vi "LSMcontroller_v65_updatedsealtest.vi"() -> ()   [LabVIEW 2015] (continued)
                                n2574 = call "tempconfigAO_seal.vi"("command"="get") -> ("Temp Config out"=w5707:T25)  [unwired: 1 in]
                                n2575 = Bundle By Name(cluster=w5707, "AO"=w5706, "E_AO"=w5705) -> (w5704:T25)
                                n2576 = call "tempconfigAO_seal.vi"("Temp Config in"=w5704, "command"="set") -> ()  [unwired: 1 out]
                                }
                                frame #1 {
                                n2577 = call "tempconfigAI_seal.vi"("command"="get") -> ("Temp Config out"=w5719:T26)  [unwired: 1 in]
                                n2578 = Unbundle By Name(w5719) -> ("AI"=w5724:refnum<k21>, "E_AI"=w5725:errorcluster)
                                n2579 = call <vilib>:"DAQmx Start Task.vi"("task/channels in"=w5724, "error in"=w5725) -> ("task out"=w5726:refnum<k21>, "error out"=w5727:errorcluster)  [unwired: 12 in]
                                n2580 = call "tempconfigAI_seal.vi"("command"="get") -> ("Temp Config out"=w5721:T26)  [unwired: 1 in]
                                n2581 = Bundle By Name(cluster=w5721, "AI"=w5726, "E_AI"=w5727) -> (w5723:T26)
                                n2582 = call "tempconfigAI_seal.vi"("Temp Config in"=w5723, "command"="set") -> ()  [unwired: 1 out]
                                }
                              }
                            }
                          }
                          n2583 = case shown="True" w5703 {
                            frame False {
                            }
                            frame True {
                              n2584 = local write "set as Rp?"(FALSE ("set as Rp?")) -> ()
                            }
                          }
                        }
                      }
                      n2585 = local read "sealtest"() -> (w5590:bool)
                      n2586 = Not(x=w5590) -> (.not. x?=w5589:bool)
                    }
                  }
                  frame #4 {
                    n2587 = call "tempconfigAO_seal.vi"("command"="get") -> ("Temp Config out"=w5754:T25)  [unwired: 1 in]
                    n2588 = Unbundle By Name(w5754) -> ("AO"=w5753:refnum<k21>[], "E_AO"=w5752:errorcluster[])
                    n2589 = call "tempconfigAI_seal.vi"("command"="get") -> ("Temp Config out"=w5741:T26)  [unwired: 1 in]
                    n2590 = call "configuration.vi"("command"="get") -> ("config out"=w5735:T11)  [unwired: 2 in, 1 out]
                    n2591 = Unbundle By Name(w5741) -> ("AI"=w5742:refnum<k21>, "E_AI"=w5743:errorcluster)
                    n2592 = Unbundle By Name(w5735) -> ("Device 1 sampleclock out"=w5732:tag, "Device 1 Starttrigger out"=w5731:tag)
                    n2593 = for {
                      tunnel: w5753 -> [w5758] mode=indexing
                      tunnel: w5752 -> [w5757] mode=indexing
                      tunnel: [w5756] -> w5748 mode=indexing
                      n2594 = call <vilib>:"DAQmx Stop Task.vi"("task/channels in"=w5758, "error in"=w5757) -> ("task out"=w5759:refnum<k21>, "error out"=w5760:errorcluster)  [unwired: 12 in]
                      n2595 = call <vilib>:"DAQmx Clear Task.vi"("task in"=w5759, "error in"=w5760) -> ("error out"=w5756:errorcluster)  [unwired: 13 in]
                    }
                    n2596 = call <vilib>:"DAQmx Stop Task.vi"("task/channels in"=w5742, "error in"=w5743) -> ("task out"=w5739:refnum<k21>, "error out"=w5738:errorcluster)  [unwired: 12 in]
                    n2597 = call <vilib>:"DAQmx Disconnect Terminals.vi"("source terminal"=tag "/Dev1/ai/SampleClock", "destination terminal"=w5732) -> ("error out"=w5729:errorcluster)  [unwired: 13 in]
                    n2598 = call <vilib>:"DAQmx Clear Task.vi"("task in"=w5739, "error in"=w5738) -> ("error out"=w5737:errorcluster)  [unwired: 13 in]
                    n2599 = call "tempconfigAO_seal.vi"("command"="get") -> ("Temp Config out"=w5749:T25)  [unwired: 1 in]
                    n2600 = Bundle By Name(cluster=w5749, "E_AO"=w5748) -> (w5747:T25)
                    n2601 = call "tempconfigAI_seal.vi"("command"="get") -> ("Temp Config out"=w5745:T26)  [unwired: 1 in]
                    n2602 = Bundle By Name(cluster=w5745, "E_AI"=w5737) -> (w5736:T26)
                    n2603 = call "tempconfigAO_seal.vi"("Temp Config in"=w5747, "command"="set") -> ()  [unwired: 1 out]
                    n2604 = call "tempconfigAI_seal.vi"("Temp Config in"=w5736, "command"="set") -> ()  [unwired: 1 out]
                    n2605 = call <vilib>:"DAQmx Disconnect Terminals.vi"("source terminal"=tag "/Dev1/ai/StartTrigger", "destination terminal"=w5731, "error in"=w5729) -> ()  [unwired: 12 in, 1 out]
                  }
                  frame #5 {
                    n2606 = call "zeropatch.vi"() -> ()  [unwired: 12 in]
                  }
                  frame #6 {
                    w5764 = T21 4 items=["no dialog", "OK message", "continue or stop message", "OK message + warnings", "continue/stop + warnings"] ("type of dialog (OK msg:1)")
                    n2607 = call "displayerrors.vi"() -> ("error IO"=w5763:errorcluster)
                    n2608 = call <vilib>:"Simple Error Handler.vi"("type of dialog (OK msg:1)"=w5764, "error in (no error)"=w5763) -> ("error out"=w5762:errorcluster)  [unwired: 3 in, 4 out]
                    n2609 = call <vilib>:"Clear Errors.vi"("error in (no error)"=w5762) -> ("error out"=w5761:errorcluster)  [unwired: 5 in, 1 out]
                    n2610 = call "seterrors.vi"("error IO"=w5761) -> ()
                  }
                }
              }
            }
          }
          event "readpatch": Value Change {
            n2611 = event-data() -> ()  [unwired: 1 in, 6 out]
            n2612 = local read "readpatch"() -> (w5765:bool)
            n2613 = case shown="True" w5765 {
              frame False {
              }
              frame True {
                n2614 = stacked-sequence {
                  seq-local: [w5766 _ _ _ _ _] -> [_ w5799 _ w5851 _ _]
                  frame #0 {
                    n2615 = stacked-sequence {
                      tunnel: [_ w5778 _] -> w5766
                      frame #0 {
                        n2616 = call "2pparameters.vi"("command"="get") -> ("params out"=w5771:T10)  [unwired: 1 in]
                        n2617 = Unbundle By Name(w5771) -> ("autoshutter"=w5772:bool)
                        n2618 = local read "OCchecked?"() -> (w5769:bool)
                        n2619 = call "sealtestwfparams.vi"("command"="set") -> ()  [unwired: 6 in, 1 out]
                        n2620 = case shown="False" w5769 {
                          frame False {
                            n2621 = One Button Dialog(message="Is the OC gain correct?", button name ("OK")="ok") -> (true=w5773:bool)
                            n2622 = local write "OCchecked?"(w5773) -> ()
                          }
                          frame True {
                          }
                        }
                        n2623 = case shown="True" w5772 {
                          frame False {
                          }
                          frame True {
                            n2624 = call "shuttercontrol.vi"("command"="close") -> ()  [unwired: 1 in, 1 out]
                          }
                        }
                        n2625 = call "allAI-temp.vi"("command"=enum16{"get", "set", "clear", "append"}."clear") -> ()  [unwired: 3 in, 2 out]
                      }
                      frame #1 {
                        n2626 = call "sealtestwfparams.vi"("command"="get") -> ("Params out"=w5784:T22)  [unwired: 6 in]
                        n2627 = Unbundle By Name(w5784) -> ("AO parameters"=w5782:T23)
                        n2628 = Index Array(array=w5782, index=1) -> (element=w5781:T24)
                        n2629 = call "generateRampedSquareWave_fromAOparameters.vi"("AO params"=w5781) -> ("Waveform"=w5777:waveform(dbl), "wflength"=w5778:i32)
                        n2630 = Build Array(w5777) -> (w5780:waveform(dbl)[])
                        n2631 = call "waveformssealtestbuffer.vi"("AO wf in"=w5780, "command"="set") -> ()  [unwired: 1 out]
                      }
                      frame #2 {
                        n2632 = local read "Vholding (mV)"() -> (w5787:sgl)
                        n2633 = local read "Current Clamp"() -> (w5793:bool)
                        n2634 = local read "Voltage Clamp"() -> (w5792:bool)
                        n2635 = local read "OCgain"() -> (w5788:sgl)
                        n2636 = local read "CC_ICgain"() -> (w5791:dbl)
                        n2637 = local read "holdon"() -> (w5786:bool)
                        n2638 = call "patchparameters.vi"("command"="get") -> ("Params out"=w5795:T13)  [unwired: 1 in]
                        n2639 = Bundle By Name(cluster=w5795, "VC"=w5792, "CC"=w5793, "CC_icg (pA/mv)"=w5791, "VC_icg (mV/mV)"=10.0, "OCG (mV/pA)"=w5788, "OVG (mV/mV)"=0.1, "Vhold (mV)"=w5787, "holdon"=w5786) -> (w5794:T13)
                        n2640 = call "patchparameters.vi"("Params in"=w5794, "command"="set") -> ()  [unwired: 1 out]
                      }
                    }
                  }
                  frame #1 {
                    w5798 = 2
                    n2641 = call "patchparameters.vi"("command"="get") -> ("Params out"=w5806:T13)  [unwired: 1 in]
                    n2642 = Unbundle By Name(w5806) -> ("holdon"=w5805:bool, "Vhold (mV)"=w5804:sgl, "CC_icg (pA/mv)"=w5812:sgl, "CC"=w5810:bool, "VC_icg (mV/mV)"=w5811:sgl)
                    n2643 = Select(t=w5812, s=w5810, f=w5811) -> (s? t:f=w5813:sgl)
                    n2644 = To Single Precision Float(number=0.001 ("y")) -> (single precision float=w5814:sgl)
                    n2645 = Compound Arithmetic op=MULTIPLY(w5804, w5813, w5814) -> (w5808:sgl)
                    n2646 = case shown="False" w5805 {
                      tunnel: w5808 -> [_ w5826]
                      tunnel: [0.0 w5826] -> w5801
                      frame False {
                      }
                      frame True {
                      }
                    }
                    n2647 = Greater Than 0?(x=w5798) -> (x > 0?=w5800:bool)
                    n2648 = case shown="True" w5800 {
                      tunnel: w5799 -> [_ w5815]
                      tunnel: w5798 -> [_ w5818]
                      frame False {
                      }
                      frame True {
                        n2649 = Initialize Array(sgl 0.0 ("element"), w5818, w5815) -> (w5816:sgl[][])
                        n2650 = call "allAI-temp.vi"("array in"=w5816, "command"=enum16{"get", "set", "clear", "append"}."set") -> ()  [unwired: 2 in, 2 out]
                      }
                    }
                    n2651 = flat-sequence {
                      tunnel: w5799 -> [w5822]
                      tunnel: w5799 -> [w5821]
                      tunnel: [w5821] -> w5803
                      tunnel: [w5820] -> w5802
                      tunnel: w5801 -> [w5820]
                      tunnel: w5803 -> [w5824]
                      tunnel: w5802 -> [w5823]
                      frame #0 {
                        n2652 = call "prepAI_sealtest.vi"("samples per channel"=w5822) -> ()  [unwired: 2 in]
                      }
                      frame #1 {
                        n2653 = call "prepAO_sealtest.vi"("Vhold"=w5823, "samples per channel"=w5824) -> ()  [unwired: 1 in]
                      }
                    }
                  }
                  frame #2 {
                    n2654 = stacked-sequence {
                      frame #0 {
                        n2655 = call "tempconfigAO.vi"("command"="get") -> ("Temp Config out"=w5830:T25)  [unwired: 1 in]
                        n2656 = Unbundle By Name(w5830) -> ("AO"=w5831:refnum<k21>[], "E_AO"=w5832:errorcluster[])
                        n2657 = for {
                          tunnel: w5831 -> [w5840] mode=indexing
                          tunnel: w5832 -> [w5839] mode=indexing
                          tunnel: [w5838] -> w5834 mode=indexing
                          tunnel: [w5837] -> w5835 mode=indexing
                          n2658 = call <vilib>:"DAQmx Start Task.vi"("task/channels in"=w5840, "error in"=w5839) -> ("task out"=w5838:refnum<k21>, "error out"=w5837:errorcluster)  [unwired: 12 in]
                        }
                        n2659 = call "tempconfigAO.vi"("command"="get") -> ("Temp Config out"=w5833:T25)  [unwired: 1 in]
                        n2660 = Bundle By Name(cluster=w5833, "AO"=w5834, "E_AO"=w5835) -> (w5836:T25)
                        n2661 = call "tempconfigAO.vi"("Temp Config in"=w5836, "command"="set") -> ()  [unwired: 1 out]
                      }
                      frame #1 {
                        n2662 = call "tempconfigAI.vi"("command"="get") -> ("Temp Config out"=w5842:T26)  [unwired: 1 in]
                        n2663 = Unbundle By Name(w5842) -> ("AI"=w5847:refnum<k21>, "E_AI"=w5848:errorcluster)
                        n2664 = call <vilib>:"DAQmx Start Task.vi"("task/channels in"=w5847, "error in"=w5848) -> ("task out"=w5849:refnum<k21>, "error out"=w5850:errorcluster)  [unwired: 12 in]
                        n2665 = call "tempconfigAI.vi"("command"="get") -> ("Temp Config out"=w5844:T26)  [unwired: 1 in]
                        n2666 = Bundle By Name(cluster=w5844, "AI"=w5849, "E_AI"=w5850) -> (w5846:T26)
                        n2667 = call "tempconfigAI.vi"("Temp Config in"=w5846, "command"="set") -> ()  [unwired: 1 out]
                      }
                    }
                  }
                  frame #3 {
                    n2668 = while {
                      tunnel: w5851 -> [w5852]
                      stop <- w5853 stop-if-true
                      n2669 = local read "readpatch"() -> (w5856:bool)
                      n2670 = Not(x=w5856) -> (.not. x?=w5855:bool)
                      n2671 = case shown="True" w5855 {
                        tunnel: w5852 -> [w5857 _]
                        frame False {
                          n2672 = stacked-sequence {
                            seq-local: [w5858 _ _ _ _ _] -> [_ w5867 _ w5890 w5937 w5956]
                            tunnel: w5857 -> [_ _ w5875 _ w5936 _]
                            frame #0 {
                              n2673 = call "patchparameters.vi"("command"="get") -> ("Params out"=w5865:T13)  [unwired: 1 in]
                              n2674 = local read "Vholding (mV)"() -> (w5862:sgl)
                              n2675 = Unbundle By Name(w5865) -> ("Vhold (mV)"=w5861:sgl, "holdon"=w5864:bool)
                              n2676 = local read "holdon"() -> (w5863:bool)
                              n2677 = Not Equal?(x=w5862, y=w5861) -> (x != y?=w5860:bool)
                              n2678 = Not Equal?(x=w5864, y=w5863) -> (x != y?=w5859:bool)
                              n2679 = Or(x=w5860, y=w5859) -> (x .or. y?=w5858:bool)
                            }
                            frame #1 {
                              n2680 = case shown="False" w5867 {
                                frame False {
                                }
                                frame True {
                                n2681 = local read "Vholding (mV)"() -> (w5870:sgl)
                                n2682 = local read "holdon"() -> (w5868:bool)
                                n2683 = call "patchparameters.vi"("command"="get") -> ("Params out"=w5871:T13)  [unwired: 1 in]
                                n2684 = Bundle By Name(cluster=w5871, "Vhold (mV)"=w5870, "holdon"=w5868) -> (w5869:T13)
                                n2685 = call "patchparameters.vi"("Params in"=w5869, "command"="set") -> ()  [unwired: 1 out]
                                }
                              }
                            }
                            frame #2 {
                              n2686 = call "tempconfigAI.vi"("command"="get") -> ("Temp Config out"=w5885:T26)  [unwired: 1 in]
                              n2687 = Unbundle By Name(w5885) -> ("AI"=w5884:refnum<k21>, "E_AI"=w5883:errorcluster)
                              n2688 = call-poly <vilib>:"DAQmx Read.vi"("task/channels in"=w5884, "number of samples per channel"=w5875, "timeout"=10.0, "error in"=w5883) -> ("task out"=w5879:refnum<k21>, "data"=w5876:i16[][], "error out"=w5888:errorcluster)  [unwired: 9 in]
                              n2689 = call "tempconfigAI.vi"("command"="get") -> ("Temp Config out"=w5880:T26)  [unwired: 1 in]
                              n2690 = Bundle By Name(cluster=w5880, "AI"=w5879, "E_AI"=w5888) -> (w5887:T26)
                              n2691 = To Single Precision Float(number=w5876) -> (single precision float=w5878:sgl[][])
                              n2692 = call "tempconfigAI.vi"("Temp Config in"=w5887, "command"="set") -> ()  [unwired: 1 out]
                              n2693 = call "allAI-temp.vi"("array in"=w5878, "command"=enum16{"get", "set", "clear", "append"}."set") -> ()  [unwired: 2 in, 2 out]
                            }
                            frame #3 {
                              n2694 = case shown="True" w5890 {
                                frame False {
                                }
                                frame True {
                                n2695 = call "tempconfigAO.vi"("command"="get") -> ("Temp Config out"=w5929:T25)  [unwired: 1 in]
                                n2696 = Unbundle By Name(w5929) -> ("AO"=w5928:refnum<k21>[], "E_AO"=w5927:errorcluster[])
                                n2697 = call "tempconfigAI.vi"("command"="get") -> ("Temp Config out"=w5916:T26)  [unwired: 1 in]
                                n2698 = Unbundle By Name(w5916) -> ("AI"=w5917:refnum<k21>, "E_AI"=w5918:errorcluster)
                                n2699 = for {
                                tunnel: w5928 -> [w5933] mode=indexing
                                tunnel: w5927 -> [w5932] mode=indexing
                                tunnel: [w5931] -> w5923 mode=indexing
                                n2700 = call <vilib>:"DAQmx Stop Task.vi"("task/channels in"=w5933, "error in"=w5932) -> ("task out"=w5934:refnum<k21>, "error out"=w5935:errorcluster)  [unwired: 12 in]
                                n2701 = call <vilib>:"DAQmx Clear Task.vi"("task in"=w5934, "error in"=w5935) -> ("error out"=w5931:errorcluster)  [unwired: 13 in]
                                }
                                n2702 = call <vilib>:"DAQmx Stop Task.vi"("task/channels in"=w5917, "error in"=w5918) -> ("task out"=w5914:refnum<k21>, "error out"=w5913:errorcluster)  [unwired: 12 in]
                                n2703 = call <vilib>:"DAQmx Clear Task.vi"("task in"=w5914, "error in"=w5913) -> ("error out"=w5912:errorcluster)  [unwired: 13 in]
                                n2704 = call "tempconfigAO.vi"("command"="get") -> ("Temp Config out"=w5924:T25)  [unwired: 1 in]
                                n2705 = Bundle By Name(cluster=w5924, "E_AO"=w5923) -> (w5922:T25)
                                n2706 = call "tempconfigAI.vi"("command"="get") -> ("Temp Config out"=w5920:T26)  [unwired: 1 in]
                                n2707 = Bundle By Name(cluster=w5920, "E_AI"=w5912) -> (w5911:T26)
                                n2708 = call "tempconfigAO.vi"("Temp Config in"=w5922, "command"="set") -> ()  [unwired: 1 out]
                                n2709 = call "tempconfigAI.vi"("Temp Config in"=w5911, "command"="set") -> ()  [unwired: 1 out]
                                }
                              }
                              n2710 = call "allAI-temp.vi"("command"=enum16{"get", "set", "clear", "append"}."get") -> ("array out"=w5894:sgl[][])  [unwired: 3 in, 1 out]
                              n2711 = call "tempconfigAI.vi"("command"="get") -> ("Temp Config out"=w5906:T26)  [unwired: 1 in]
                              n2712 = call "tempconfigAI.vi"("command"="get") -> ("Temp Config out"=w5908:T26)  [unwired: 1 in]
                              n2713 = Unbundle By Name(w5906) -> ("header"=w5904:dbl[])
                              n2714 = Unbundle By Name(w5908) -> ("header"=w5910:dbl[])
                              n2715 = Index Array(array=w5894, index (row) #1=1 ("index (row)"), index (row) #2=0 ("index (row)")) -> (element #1=w5892:sgl[], element #2=w5891:sgl[])  [unwired: 2 in]
                              n2716 = local read "OCgain"() -> (w5898:sgl)
                              n2717 = call "Unscaledtoscaled.vi"("Unscaled Data"=w5892, "Header Information"=w5904) -> ("Array"=w5903:sgl[])  [unwired: 1 in]
                              n2718 = call "Unscaledtoscaled.vi"("Unscaled Data"=w5891, "Header Information"=w5910) -> ("Array"=w5907:sgl[])  [unwired: 1 in]
                              n2719 = Multiply(x=w5903, y=0.1) -> (x*y=w5900:dbl[])
                              n2720 = Divide(x=w5907, y=w5898) -> (x/y=w5899:sgl[])
                              n2721 = Build Array(w5900, w5899) -> (w5902:dbl[][])
                              n2722 = Multiply(x=w5902, y=1000.0) -> (x*y=w5889:dbl[][])
                              n2723 = local write "Patch readout"(w5889) -> ()
                            }
                            frame #4 {
                              n2724 = case shown="True" w5937 {
                                tunnel: w5936 -> [_ w5938]
                                frame False {
                                }
                                frame True {
                                n2725 = call "patchparameters.vi"("command"="get") -> ("Params out"=w5942:T13)  [unwired: 1 in]
                                n2726 = Unbundle By Name(w5942) -> ("holdon"=w5941:bool, "Vhold (mV)"=w5940:sgl, "CC_icg (pA/mv)"=w5948:sgl, "CC"=w5946:bool, "VC_icg (mV/mV)"=w5947:sgl)
                                n2727 = Select(t=w5948, s=w5946, f=w5947) -> (s? t:f=w5949:sgl)
                                n2728 = To Single Precision Float(number=0.001 ("y")) -> (single precision float=w5950:sgl)
                                n2729 = Compound Arithmetic op=MULTIPLY(w5940, w5949, w5950) -> (w5944:sgl)
                                n2730 = case shown="True" w5941 {
                                tunnel: w5944 -> [_ w5955]
                                tunnel: [0.0 w5955] -> w5939
                                frame False {
                                }
                                frame True {
                                }
                                }
                                n2731 = flat-sequence {
                                tunnel: w5938 -> [w5951]
                                tunnel: w5939 -> [w5953]
                                tunnel: w5938 -> [w5952]
                                frame #0 {
                                n2732 = call "prepAI_sealtest.vi"("samples per channel"=w5951) -> ()  [unwired: 2 in]
                                }
                                frame #1 {
                                n2733 = call "prepAO_sealtest.vi"("Vhold"=w5953, "samples per channel"=w5952) -> ()  [unwired: 1 in]
                                }
                                }
                                }
                              }
                            }
                            frame #5 {
                              n2734 = case shown="True" w5956 {
                                frame False {
                                }
                                frame True {
                                n2735 = stacked-sequence {
                                frame #0 {
                                n2736 = call "tempconfigAO.vi"("command"="get") -> ("Temp Config out"=w5963:T25)  [unwired: 1 in]
                                n2737 = Unbundle By Name(w5963) -> ("AO"=w5962:refnum<k21>[], "E_AO"=w5961:errorcluster[])
                                n2738 = for {
                                tunnel: w5962 -> [w5970] mode=indexing
                                tunnel: w5961 -> [w5969] mode=indexing
                                tunnel: [w5968] -> w5959 mode=indexing
                                tunnel: [w5967] -> w5958 mode=indexing
                                n2739 = call <vilib>:"DAQmx Start Task.vi"("task/channels in"=w5970, "error in"=w5969) -> ("task out"=w5968:refnum<k21>, "error out"=w5967:errorcluster)  [unwired: 12 in]
                                }
                                n2740 = call "tempconfigAO.vi"("command"="get") -> ("Temp Config out"=w5960:T25)  [unwired: 1 in]
                                n2741 = Bundle By Name(cluster=w5960, "AO"=w5959, "E_AO"=w5958) -> (w5957:T25)
                                n2742 = call "tempconfigAO.vi"("Temp Config in"=w5957, "command"="set") -> ()  [unwired: 1 out]
                                }
                                frame #1 {
                                n2743 = call "tempconfigAI.vi"("command"="get") -> ("Temp Config out"=w5972:T26)  [unwired: 1 in]
                                n2744 = Unbundle By Name(w5972) -> ("AI"=w5977:refnum<k21>, "E_AI"=w5978:errorcluster)
                                n2745 = call <vilib>:"DAQmx Start Task.vi"("task/channels in"=w5977, "error in"=w5978) -> ("task out"=w5979:refnum<k21>, "error out"=w5980:errorcluster)  [unwired: 12 in]
                                n2746 = call "tempconfigAI.vi"("command"="get") -> ("Temp Config out"=w5974:T26)  [unwired: 1 in]
                                n2747 = Bundle By Name(cluster=w5974, "AI"=w5979, "E_AI"=w5980) -> (w5976:T26)
                                n2748 = call "tempconfigAI.vi"("Temp Config in"=w5976, "command"="set") -> ()  [unwired: 1 out]
                                }
                                }
                                }
                              }
                            }
                          }
                        }
                        frame True {
                        }
                      }
                      n2749 = local read "readpatch"() -> (w5854:bool)
                      n2750 = Not(x=w5854) -> (.not. x?=w5853:bool)
                    }
                  }
                  frame #4 {
                    n2751 = call "tempconfigAO.vi"("command"="get") -> ("Temp Config out"=w6006:T25)  [unwired: 1 in]
                    n2752 = Unbundle By Name(w6006) -> ("AO"=w6005:refnum<k21>[], "E_AO"=w6004:errorcluster[])
                    n2753 = call "configuration.vi"("command"="get") -> ("config out"=w5987:T11)  [unwired: 2 in, 1 out]
                    n2754 = call "tempconfigAI.vi"("command"="get") -> ("Temp Config out"=w5993:T26)  [unwired: 1 in]
                    n2755 = Unbundle By Name(w5987) -> ("Device 1 sampleclock out"=w5984:tag, "Device 1 Starttrigger out"=w5983:tag)
                    n2756 = Unbundle By Name(w5993) -> ("AI"=w5994:refnum<k21>, "E_AI"=w5995:errorcluster)
                    n2757 = for {
                      tunnel: w6005 -> [w6010] mode=indexing
                      tunnel: w6004 -> [w6009] mode=indexing
                      tunnel: [w6008] -> w6000 mode=indexing
                      n2758 = call <vilib>:"DAQmx Stop Task.vi"("task/channels in"=w6010, "error in"=w6009) -> ("task out"=w6011:refnum<k21>, "error out"=w6012:errorcluster)  [unwired: 12 in]
                      n2759 = call <vilib>:"DAQmx Clear Task.vi"("task in"=w6011, "error in"=w6012) -> ("error out"=w6008:errorcluster)  [unwired: 13 in]
                    }
                    n2760 = call <vilib>:"DAQmx Stop Task.vi"("task/channels in"=w5994, "error in"=w5995) -> ("task out"=w5991:refnum<k21>, "error out"=w5990:errorcluster)  [unwired: 12 in]
                    n2761 = call <vilib>:"DAQmx Disconnect Terminals.vi"("source terminal"=tag "/Dev1/ai/SampleClock", "destination terminal"=w5984) -> ("error out"=w5981:errorcluster)  [unwired: 13 in]
                    n2762 = call <vilib>:"DAQmx Clear Task.vi"("task in"=w5991, "error in"=w5990) -> ("error out"=w5989:errorcluster)  [unwired: 13 in]
                    n2763 = call "tempconfigAO.vi"("command"="get") -> ("Temp Config out"=w6001:T25)  [unwired: 1 in]
                    n2764 = Bundle By Name(cluster=w6001, "E_AO"=w6000) -> (w5999:T25)
                    n2765 = call "tempconfigAI.vi"("command"="get") -> ("Temp Config out"=w5997:T26)  [unwired: 1 in]
                    n2766 = Bundle By Name(cluster=w5997, "E_AI"=w5989) -> (w5988:T26)
                    n2767 = call "tempconfigAO.vi"("Temp Config in"=w5999, "command"="set") -> ()  [unwired: 1 out]
                    n2768 = call <vilib>:"DAQmx Disconnect Terminals.vi"("source terminal"=tag "/Dev1/ai/StartTrigger", "destination terminal"=w5983, "error in"=w5981) -> ()  [unwired: 12 in, 1 out]
                    n2769 = call "tempconfigAI.vi"("Temp Config in"=w5988, "command"="set") -> ()  [unwired: 1 out]
                  }
                  frame #5 {
                    w6015 = T21 4 items=["no dialog", "OK message", "continue or stop message", "OK message + warnings", "continue/stop + warnings"] ("type of dialog (OK msg:1)")
                    n2770 = call "displayerrors.vi"() -> ("error IO"=w6014:errorcluster)
                    n2771 = call "zeropatch.vi"() -> ()  [unwired: 12 in]
                    n2772 = call <vilib>:"Simple Error Handler.vi"("type of dialog (OK msg:1)"=w6015, "error in (no error)"=w6014) -> ("error out"=w6013:errorcluster)  [unwired: 3 in, 4 out]
                    n2773 = call <vilib>:"Clear Errors.vi"("error in (no error)"=w6013) -> ()  [unwired: 5 in, 2 out]
                  }
                }
              }
            }
          }
          event "Current Clamp": Value Change {
            n2774 = event-data() -> ()  [unwired: 1 in, 6 out]
            n2775 = local read "Current Clamp"() -> (w6020:bool)
            n2776 = property on="Vholding (mV)" class="DigNum (strict)"("Caption.Text"="Ihold (pA)") -> ()  [unwired: 2 in, 2 out]
            n2777 = Not(x=w6020) -> (.not. x?=w6019:bool)
            n2778 = property on="Voltage Clamp" class="Bool (strict)"("Value"=w6019) -> ()  [unwired: 2 in, 2 out]
            n2779 = One Button Dialog(message="Have you switched the HEKA to CC and changed the external input cable?", button name ("OK")="Ok") -> ()  [unwired: 1 out]
          }
          event "Voltage Clamp": Value Change {
            n2780 = event-data() -> ()  [unwired: 1 in, 6 out]
            n2781 = local read "Voltage Clamp"() -> (w6025:bool)
            n2782 = Not(x=w6025) -> (.not. x?=w6024:bool)
            n2783 = property on="Current Clamp" class="Bool (strict)"("Value"=w6024) -> ()  [unwired: 2 in, 2 out]
            n2784 = One Button Dialog(message="Have you switched the HEKA to VC and changed the external input cable?", button name ("OK")="Ok") -> ()  [unwired: 1 out]
            n2785 = property on="Vholding (mV)" class="DigNum (strict)"("Caption.Text"="Vhold (mV)") -> ()  [unwired: 2 in, 2 out]
          }
          event "OCgain": Value Change {
            n2786 = event-data() -> ()  [unwired: 1 in, 6 out]
            n2787 = local read "OCgain"() -> (w6028:sgl)
            n2788 = Less?(x=w6028, y=0.3) -> (x < y?=w6026:bool)
            n2789 = case shown="True" w6026 {
              frame False {
                w6029 = 10.0 items=["0.1"=10.0, "10"=0.1] ("CC_ICgain")
                n2790 = local write "CC_ICgain"(w6029) -> ()
              }
              frame True {
                w6030 = 0.1 items=["0.1"=10.0, "10"=0.1] ("CC_ICgain")
                n2791 = local write "CC_ICgain"(w6030) -> ()
              }
            }
          }
          event "holdon": Value Change {
            n2792 = event-data() -> ()  [unwired: 1 in, 6 out]
            n2793 = stacked-sequence {
              frame #0 {
                n2794 = local read "Vholding (mV)"() -> (w6034:sgl)
                n2795 = local read "holdon"() -> (w6031:bool)
                n2796 = call "patchparameters.vi"("command"="get") -> ("Params out"=w6035:T13)  [unwired: 1 in]
                n2797 = Bundle By Name(cluster=w6035, "Vhold (mV)"=w6034, "holdon"=w6031) -> (w6032:T13)
                n2798 = call "patchparameters.vi"("Params in"=w6032, "command"="set") -> ()  [unwired: 1 out]
              }
              frame #1 {
                n2799 = call "zeropatch.vi"() -> ()  [unwired: 12 in]
              }
            }
          }
          event "Vholding (mV)": Value Change {
            n2800 = event-data() -> ()  [unwired: 1 in, 6 out]
            n2801 = local read "holdon"() -> (w6037:bool)
            n2802 = case shown="True" w6037 {
              frame False {
              }
              frame True {
                n2803 = stacked-sequence {
                  frame #0 {
                    n2804 = local read "Vholding (mV)"() -> (w6040:sgl)
                    n2805 = local read "holdon"() -> (w6041:bool)
                    n2806 = call "patchparameters.vi"("command"="get") -> ("Params out"=w6042:T13)  [unwired: 1 in]
                    n2807 = Bundle By Name(cluster=w6042, "Vhold (mV)"=w6040, "holdon"=w6041) -> (w6038:T13)
                    n2808 = call "patchparameters.vi"("Params in"=w6038, "command"="set") -> ()  [unwired: 1 out]
                  }
                  frame #1 {
                    n2809 = call "zeropatch.vi"() -> ()  [unwired: 12 in]
                  }
                }
              }
            }
          }
          event "AI channels": Value Change {
            n2810 = event-data() -> ()  [unwired: 1 in, 6 out]
            n2811 = local read "CI channels"() -> (w6051:i32[])
            n2812 = local read "AI channels"() -> (w6052:i32[])
            n2813 = call "configuration.vi"("command"="get") -> ("config out"=w6045:T11)  [unwired: 2 in, 1 out]
            n2814 = Unbundle By Name(w6045) -> ("CI names"=w6046:string[], "AI names"=w6047:string[])
            n2815 = for {
              tunnel: w6051 -> [w6057] mode=indexing
              tunnel: w6046 -> [w6058]
              tunnel: [w6056] -> w6048 mode=indexing
              n2816 = Index Array(array=w6058, index=w6057) -> (element=w6056:string)
            }
            n2817 = for {
              tunnel: w6052 -> [w6054] mode=indexing
              tunnel: w6047 -> [w6055]
              tunnel: [w6053] -> w6049 mode=indexing
              n2818 = Index Array(array=w6055, index=w6054) -> (element=w6053:string)
            }
            n2819 = Build Array (concatenate)(w6048, w6049) -> (w6050:string[])
            n2820 = property on="image1list" class="Ring (strict)"("Strings []"=w6050) -> ()  [unwired: 2 in, 2 out]
            n2821 = property on="image2list" class="Ring (strict)"("Strings []"=w6050) -> ()  [unwired: 2 in, 2 out]
          }
          event "CI channels": Value Change {
            n2822 = event-data() -> ()  [unwired: 1 in, 6 out]
            n2823 = local read "CI channels"() -> (w6066:i32[])
            n2824 = local read "AI channels"() -> (w6067:i32[])
            n2825 = call "configuration.vi"("command"="get") -> ("config out"=w6060:T11)  [unwired: 2 in, 1 out]
            n2826 = Unbundle By Name(w6060) -> ("CI names"=w6061:string[], "AI names"=w6062:string[])
            n2827 = for {
              tunnel: w6066 -> [w6072] mode=indexing
              tunnel: w6061 -> [w6073]
              tunnel: [w6071] -> w6063 mode=indexing
              n2828 = Index Array(array=w6073, index=w6072) -> (element=w6071:string)
            }
            n2829 = for {
              tunnel: w6067 -> [w6069] mode=indexing
              tunnel: w6062 -> [w6070]
              tunnel: [w6068] -> w6064 mode=indexing
              n2830 = Index Array(array=w6070, index=w6069) -> (element=w6068:string)
            }
            n2831 = Build Array (concatenate)(w6063, w6064) -> (w6065:string[])
            n2832 = property on="image1list" class="Ring (strict)"("Strings []"=w6065) -> ()  [unwired: 2 in, 2 out]
            n2833 = property on="image2list" class="Ring (strict)"("Strings []"=w6065) -> ()  [unwired: 2 in, 2 out]
          }
          event "setdatdir": Value Change {
            n2834 = event-data() -> ()  [unwired: 1 in, 5 out]
            n2835 = case shown="True" "setdatdir" {
              frame False {
              }
              frame True {
                n2836 = stacked-sequence {
                  frame #0 {
                    n2837 = local read "data dir"() -> (w6075:path)
                    n2838 = call "File Dialog"("start path"=w6075, "prompt"="Please select data directory...") -> ("selected path"=w6077:path, "cancelled"=w6076:bool, "error out"=w6078:errorcluster)  [unwired: 10 in, 1 out]
                    n2839 = case shown="False" w6076 {
                      tunnel: w6077 -> [w6086 _]
                      tunnel: w6078 -> [w6083 w6089]
                      tunnel: [w6081 w6089] -> w6080
                      frame False {
                        n2840 = local write "data dir"(w6086) -> ()
                        n2841 = call "configuration.vi"("error in"=w6083, "command"="get") -> ("Error out"=w6082:errorcluster, "config out"=w6088:T11)  [unwired: 1 in]
                        n2842 = Bundle By Name(cluster=w6088, "master data dir"=w6086) -> (w6087:T11)
                        n2843 = call "configuration.vi"("error in"=w6082, "config in"=w6087, "command"="set") -> ("Error out"=w6081:errorcluster)  [unwired: 1 out]
                      }
                      frame True {
                      }
                    }
                    n2844 = local write "status"(w6080) -> ()
                  }
                  frame #1 {
                    n2845 = property on="setdatdir" class="Bool (strict)"("Value"=FALSE ("setdatdir")) -> ()  [unwired: 2 in, 2 out]
                  }
                }
              }
            }
          }
          event "Shutter": Value Change {
            n2846 = event-data() -> ()  [unwired: 1 in, 5 out]
            n2847 = case shown="False" "Shutter" {
              frame False {
                n2848 = call "shuttercontrol.vi"("command"="close") -> ()  [unwired: 1 in, 1 out]
              }
              frame True {
                n2849 = call "shuttercontrol.vi"("command"="open") -> ()  [unwired: 1 in, 1 out]
              }
            }
          }
          event "ROI": Value Change {
            n2850 = event-data() -> ()  [unwired: 1 in, 5 out]
            n2851 = local read "ROI"() -> (w6094:bool)
            n2852 = case shown="True" w6094 {
              frame False {
              }
              frame True {
                n2853 = stacked-sequence {
                  frame #0 {
                    n2854 = local read "Square pixels"() -> (w6111:bool)
                    n2855 = local read "square matrix"() -> (w6110:bool)
                    n2856 = local read "Vx-max ref"() -> (w6116:dbl)
                    n2857 = local read "Vx-min ref"() -> (w6115:dbl)
                    n2858 = local read "Vy-min ref"() -> (w6112:dbl)
                    n2859 = local read "ypixels ref"() -> (w6114:i32)
                    n2860 = local read "Vy-max ref"() -> (w6113:dbl)
                    n2861 = local read "xpixels ref"() -> (w6117:i32)
                    n2862 = local read "Angle ref"() -> (w6109:dbl)
                    n2863 = local read "Colormap"() -> (w6118:i32)
                    n2864 = call "2pparameters.vi"("command"="get") -> ("params out"=w6121:T10)  [unwired: 1 in]
                    n2865 = Bundle By Name(cluster=w6121, "Xpixels Img"=w6117, "Vx-min Img"=w6115, "VX-max Img"=w6116, "Ypixels Img"=w6114, "Vy-min Img"=w6112, "Vy-max Img"=w6113, "Colormap"=w6118, "square pixels"=w6111, "square matrix"=w6110, "Angle Img"=w6109) -> (w6120:T10)
                    n2866 = call "2pparameters.vi"("Params in"=w6120, "command"="set") -> ()  [unwired: 1 out]
                    n2867 = local read "Vx-max draw"() -> (w6101:dbl)
                    n2868 = local read "Angle drawing"() -> (w6108:dbl)
                    n2869 = local read "Vx-min draw"() -> (w6102:dbl)
                    n2870 = local read "Vy-min draw"() -> (w6105:dbl)
                    n2871 = local read "ypixels draw"() -> (w6103:dbl)
                    n2872 = local read "Vy-max draw"() -> (w6104:dbl)
                    n2873 = local read "Square pixels"() -> (w6106:bool)
                    n2874 = local read "square matrix"() -> (w6107:bool)
                    n2875 = local read "xpixels draw"() -> (w6100:dbl)
                    n2876 = local read "Colormap"() -> (w6099:i32)
                    n2877 = call "2pparameters.vi"("command"="get") -> ("params out"=w6096:T10)  [unwired: 1 in]
                    n2878 = Bundle By Name(cluster=w6096, "Xpixels"=w6100, "Vxminref"=w6102, "Vxmaxref"=w6101, "Ypixels"=w6103, "Vyminref"=w6105, "Vymaxref"=w6104, "Colormap"=w6099, "square pixels"=w6106, "square matrix"=w6107, "Angle draw"=w6108) -> (w6097:T10)
                    n2879 = call "2pparameters.vi"("Params in"=w6097, "command"="set") -> ()  [unwired: 1 out]
                  }
                  frame #1 {
                    n2880 = Current VI's Path() -> (path=w6132:path)
                    n2881 = Strip Path(path=w6132) -> (stripped path=w6133:path)  [unwired: 1 out]
                    n2882 = Build Path(base path=w6133, name or relative path="subVIs\\Image\\SetROI_v4.vi") -> (appended path=w6131:path)
                    n2883 = call <vilib>:"Set Busy.vi"() -> ("error out"=w6129:errorcluster)  [unwired: 10 in, 1 out]
                    n2884 = Open VI Reference(type specifier VI Refnum (for type only)=refnum<vi> refnum, vi path=w6131, error in (no error)=w6129) -> (vi reference=w6127:refnum<vi>, error out=w6125:errorcluster)  [unwired: 3 in]
                    n2885 = call-by-ref "?"(reference=w6127, error in=w6125) -> (reference out=w6126:refnum<vi>, error out=w6124:errorcluster)  [unwired: 1 in]
                    n2886 = Close Reference(reference=w6126, error in (no error)=w6124) -> (error out=w6128:errorcluster)
                    n2887 = call <vilib>:"Unset Busy.vi"("error in (no error)"=w6128) -> ()  [unwired: 10 in, 1 out]
                    n2888 = local write "status"(w6128) -> ()
                  }
                  frame #2 {
                    n2889 = call "2pparameters.vi"("command"="get") -> ("params out"=w6158:T10)  [unwired: 1 in]
                    n2890 = Unbundle By Name(w6158) -> ("Xpixels Img"=w6157:i32, "Vx-min Img"=w6156:dbl, "VX-max Img"=w6155:dbl, "Ypixels Img"=w6154:i32, "Vy-min Img"=w6153:dbl, "Vy-max Img"=w6152:dbl, "Colormap"=w6151:u16, "square pixels"=w6150:bool, "square matrix"=w6149:bool, "Angle Img"=w6148:dbl, "Drawing Mode"=w6147:u16)
                    n2891 = local write "xpixels ref"(w6157) -> ()
                    n2892 = local write "Vx-min ref"(w6156) -> ()
                    n2893 = local write "Vx-max ref"(w6155) -> ()
                    n2894 = local write "ypixels ref"(w6154) -> ()
                    n2895 = local write "Vy-min ref"(w6153) -> ()
                    n2896 = local write "Vy-max ref"(w6152) -> ()
                    n2897 = local write "Colormap"(w6151) -> ()
                    n2898 = local write "Square pixels"(w6150) -> ()
                    n2899 = local write "square matrix"(w6149) -> ()
                    n2900 = local write "Angle ref"(w6148) -> ()
                    n2901 = local write "ROI Type"(w6147) -> ()
                    n2902 = call "2pparameters.vi"("command"="get") -> ("params out"=w6141:T10)  [unwired: 1 in]
                    n2903 = Unbundle By Name(w6141) -> ("Xpixels"=w6135:i32, "Vxminref"=w6139:dbl, "Vxmaxref"=w6138:dbl, "Ypixels"=w6134:i32, "Vyminref"=w6137:dbl, "Vymaxref"=w6136:dbl, "Colormap"=w6142:u16, "square pixels"=w6143:bool, "square matrix"=w6144:bool, "Angle draw"=w6145:dbl, "Drawing Mode"=w6146:u16)
                    n2904 = local write "Vy-max draw"(w6136) -> ()
                    n2905 = local write "Angle drawing"(w6145) -> ()
                    n2906 = local write "Colormap"(w6142) -> ()
                    n2907 = local write "Square pixels"(w6143) -> ()
                    n2908 = local write "square matrix"(w6144) -> ()
                    n2909 = local write "ROI Type"(w6146) -> ()
                    n2910 = local write "xpixels draw"(w6135) -> ()
                    n2911 = local write "ypixels draw"(w6134) -> ()
                    n2912 = local write "Vx-min draw"(w6139) -> ()
                    n2913 = local write "Vx-max draw"(w6138) -> ()
                    n2914 = local write "Vy-min draw"(w6137) -> ()
                  }
                  frame #3 {
                    n2915 = property on="ROI" class="Bool (strict)"("Val(Sgnl)"=FALSE ("x/y scan")) -> ()  [unwired: 2 in, 2 out]
                  }
                }
              }
            }
          }
          event "Xdattype": Value Change {
            n2916 = event-data() -> ()  [unwired: 1 in, 1 out]
            n2917 = case shown="True" "Xdattype" {
              frame False {
              }
              frame True {
                n2918 = stacked-sequence {
                  frame #0 {
                    n2919 = Current VI's Path() -> (path=w6171:path)
                    n2920 = Strip Path(path=w6171) -> (stripped path=w6172:path)  [unwired: 1 out]
                    n2921 = Build Path(base path=w6172, name or relative path="subVIs\\Misc\\Changedataconfig.vi") -> (appended path=w6170:path)
                    n2922 = call <vilib>:"Set Busy.vi"() -> ("error out"=w6168:errorcluster)  [unwired: 10 in, 1 out]
                    n2923 = Open VI Reference(type specifier VI Refnum (for type only)=refnum<vi> refnum, vi path=w6170, error in (no error)=w6168) -> (vi reference=w6163:refnum<vi>, error out=w6165:errorcluster)  [unwired: 3 in]
                    n2924 = call-by-ref "?"(reference=w6163, error in=w6165) -> (reference out=w6167:refnum<vi>, error out=w6166:errorcluster)  [unwired: 12 in]
                    n2925 = Close Reference(reference=w6167, error in (no error)=w6166) -> (error out=w6162:errorcluster)
                    "status" <- w6162
                    n2926 = call <vilib>:"Unset Busy.vi"("error in (no error)"=w6162) -> ()  [unwired: 10 in, 1 out]
                  }
                  frame #1 {
                    n2927 = property on="Xdattype" class="Bool (strict)"("Val(Sgnl)"=FALSE ("x/y scan")) -> ()  [unwired: 2 in, 2 out]
                  }
                }
              }
            }
          }
          event "XautoOD": Value Change {
            n2928 = event-data() -> ()  [unwired: 1 in, 1 out]
            n2929 = case shown="True" "XautoOD" {
              frame False {
              }
              frame True {
                n2930 = stacked-sequence {
                  frame #0 {
                    n2931 = Current VI's Path() -> (path=w6184:path)
                    n2932 = Strip Path(path=w6184) -> (stripped path=w6185:path)  [unwired: 1 out]
                    n2933 = Build Path(base path=w6185, name or relative path="subVIs\\Misc\\ChangeautoODs.vi") -> (appended path=w6183:path)
                    n2934 = call <vilib>:"Set Busy.vi"() -> ("error out"=w6181:errorcluster)  [unwired: 10 in, 1 out]
                    n2935 = Open VI Reference(type specifier VI Refnum (for type only)=refnum<vi> refnum, vi path=w6183, error in (no error)=w6181) -> (vi reference=w6176:refnum<vi>, error out=w6178:errorcluster)  [unwired: 3 in]
                    n2936 = call-by-ref "?"(reference=w6176, error in=w6178) -> (reference out=w6180:refnum<vi>, error out=w6179:errorcluster)  [unwired: 12 in]
                    n2937 = Close Reference(reference=w6180, error in (no error)=w6179) -> (error out=w6175:errorcluster)
                    "status 2" <- w6175
                    n2938 = call <vilib>:"Unset Busy.vi"("error in (no error)"=w6175) -> ()  [unwired: 10 in, 1 out]
                  }
                  frame #1 {
                    n2939 = property on="XautoOD" class="Bool (strict)"("Val(Sgnl)"=FALSE ("x/y scan")) -> ()  [unwired: 2 in, 2 out]
                  }
                }
              }
            }
          }
          event "SetMan": Value Change {
            n2940 = event-data() -> ()  [unwired: 1 in, 1 out]
            n2941 = case shown="True" "SetMan" {
              frame False {
              }
              frame True {
                n2942 = stacked-sequence {
                  frame #0 {
                    w6188 = u16 0 items=["Rectangle", "Circle", "Freeform Boundary", "Freeform Interior"] ("ROI Type")
                    n2943 = local write "ROI Type"(w6188) -> ()
                    n2944 = local read "Square pixels"() -> (w6194:bool)
                    n2945 = case shown="True" w6194 {
                      frame False {
                        n2946 = local read "square matrix"() -> (w6195:bool)
                        n2947 = case shown="False" w6195 {
                          frame False {
                            "ypixels ref" <- "ypixels"
                            "xpixels ref" <- "xpixels"
                          }
                          frame True {
                            n2948 = local read "xpixels"() -> (w6200:i32)
                            n2949 = local read "ypixels"() -> (w6199:i32)
                            n2950 = Max & Min(x=w6200, y=w6199) -> (max(x,y)=w6198:i32)  [unwired: 1 out]
                            n2951 = local write "xpixels ref"(w6198) -> ()
                            n2952 = local write "ypixels ref"(w6198) -> ()
                          }
                        }
                      }
                      frame True {
                        n2953 = local read "square matrix"() -> (w6201:bool)
                        n2954 = case shown="False" w6201 {
                          frame False {
                            n2955 = local read "Vxmax"() -> (w6215:dbl)
                            n2956 = local read "Vx-min"() -> (w6214:dbl)
                            n2957 = local read "Vy-max"() -> (w6210:dbl)
                            n2958 = local read "Vy-min"() -> (w6211:dbl)
                            n2959 = Subtract(x=w6210, y=w6211) -> (x-y=w6212:dbl)
                            n2960 = Subtract(x=w6215, y=w6214) -> (x-y=w6213:dbl)
                            n2961 = Absolute Value(x=w6212) -> (abs(x)=w6203:dbl)
                            n2962 = Absolute Value(x=w6213) -> (abs(x)=w6204:dbl)
                            n2963 = Divide(x=w6204, y=w6203) -> (x/y=w6209:dbl)
                            n2964 = Greater Or Equal?(x=w6204, y=w6203) -> (x >= y?=w6202:bool)
                            n2965 = local read "xpixels"() -> (w6208:i32)
                            n2966 = local read "ypixels"() -> (w6205:i32)
                            n2967 = case shown="False" w6202 {
                              tunnel: w6209 -> [w6220 w6223]
                              tunnel: w6208 -> [w6217 _]
                              tunnel: [w6217 w6222] -> w6207
                              tunnel: [w6216 w6221] -> w6206
                              tunnel: w6205 -> [_ w6221]
                              frame False {
                                n2968 = To Double Precision Float(number=w6217) -> (double precision float=w6219:dbl)
                                n2969 = Divide(x=w6219, y=w6220) -> (x/y=w6218:dbl)
                                n2970 = To Long Integer(number=w6218) -> (32bit integer=w6216:i32)
                              }
                              frame True {
                                n2971 = To Double Precision Float(number=w6221) -> (double precision float=w6225:dbl)
                                n2972 = Multiply(x=w6225, y=w6223) -> (x*y=w6224:dbl)
                                n2973 = To Long Integer(number=w6224) -> (32bit integer=w6222:i32)
                              }
                            }
                            n2974 = local write "ypixels ref"(w6206) -> ()
                            n2975 = local write "xpixels ref"(w6207) -> ()
                          }
                          frame True {
                          }
                        }
                      }
                    }
                    "Vx-max ref" <- "Vxmax"
                    "Vx-min ref" <- "Vx-min"
                    "Vy-max ref" <- "Vy-max"
                    "Vy-min ref" <- "Vy-min"
                    "Angle ref" <- "Angle"
                  }
                  frame #1 {
                    n2976 = property on="SetMan" class="Bool (strict)"("Val(Sgnl)"=FALSE ("Value (Signaling)")) -> ()  [unwired: 2 in, 2 out]
                  }
                }
              }
            }
          }
          event "SetMan 2": Value Change {
            n2977 = event-data() -> ()  [unwired: 1 in, 1 out]
            n2978 = case shown="True" "SetMan 2" {
              frame False {
              }
              frame True {
                n2979 = stacked-sequence {
                  frame #0 {
                    n2980 = local write "Vx-ref"("Vx") -> ()
                    n2981 = local write "Vy-ref"("Vy") -> ()
                  }
                  frame #1 {
                    n2982 = property on="SetMan 2" class="Bool (strict)"("Val(Sgnl)"=FALSE ("Value (Signaling)")) -> ()  [unwired: 2 in, 2 out]
                  }
                }
              }
            }
          }
          event "Reset Coords": Value Change {
            n2983 = event-data() -> ("NewVal"=w6231:bool)  [unwired: 1 in, 5 out]
            n2984 = case shown="True" w6231 {
              frame False {
              }
              frame True {
                n2985 = stacked-sequence {
                  frame #0 {
                    n2986 = local write "xpixels"(256 ("xpixels")) -> ()
                    n2987 = local write "ypixels"(256 ("ypixels")) -> ()
                    n2988 = local write "Vxmax"(9.0 ("Vx-max")) -> ()
                    n2989 = local write "Vx-min"(-9.0 ("Vx-min")) -> ()
                    n2990 = local write "Vy-max"(9.0 ("Vy-max")) -> ()
                    n2991 = local write "Vy-min"(-9.0 ("Vy-min")) -> ()
                    n2992 = local write "Angle"(0.0 ("Angle")) -> ()
                  }
                  frame #1 {
                    n2993 = property on="Reset Coords" class="Bool (strict)"("Value"=FALSE ("TROI")) -> ()  [unwired: 2 in, 2 out]
                  }
                }
              }
            }
          }
          event "TROI": Value Change {
            n2994 = event-data() -> ()  [unwired: 1 in, 1 out]
            n2995 = case shown="True" "TROI" {
              frame False {
              }
              frame True {
                n2996 = stacked-sequence {
                  frame #0 {
                    n2997 = local read "Vy-min ref"() -> (w6245:dbl)
                    n2998 = local read "Vy-max ref"() -> (w6244:dbl)
                    n2999 = local read "Vx-max ref"() -> (w6242:dbl)
                    n3000 = local read "Vx-min ref"() -> (w6243:dbl)
                    n3001 = local read "ypixels ref"() -> (w6247:i32)
                    n3002 = local read "xpixels ref"() -> (w6246:i32)
                    n3003 = local read "Angle ref"() -> (w6241:dbl)
                    n3004 = local write "Angle"(w6241) -> ()
                    n3005 = local write "xpixels"(w6246) -> ()
                    n3006 = local write "Vy-min"(w6245) -> ()
                    n3007 = local write "Vy-max"(w6244) -> ()
                    n3008 = local write "Vx-min"(w6243) -> ()
                    n3009 = local write "ypixels"(w6247) -> ()
                    n3010 = local write "Vxmax"(w6242) -> ()
                  }
                  frame #1 {
                    n3011 = property on="TROI" class="Bool (strict)"("Value"=FALSE ("TROI")) -> ()  [unwired: 2 in, 2 out]
                  }
                }
              }
            }
          }
          event "TROI 2": Value Change {
            n3012 = event-data() -> ()  [unwired: 1 in, 1 out]
            n3013 = case shown="True" "TROI 2" {
              frame False {
              }
              frame True {
                n3014 = stacked-sequence {
                  frame #0 {
                    n3015 = local read "Vx-ref"() -> (w6250:dbl)
                    n3016 = local read "Vy-ref"() -> (w6251:dbl)
                    n3017 = local write "Vx"(w6250) -> ()
                    n3018 = local write "Vy"(w6251) -> ()
                  }
                  frame #1 {
                    n3019 = property on="TROI 2" class="Bool (strict)"("Value"=FALSE ("TROI")) -> ()  [unwired: 2 in, 2 out]
                  }
                }
              }
            }
          }
          event "Square pixels": Value Change {
            n3020 = event-data() -> ()  [unwired: 1 in, 1 out]
            n3021 = case shown="True" "Square pixels" {
              frame False {
              }
              frame True {
                n3022 = property on="square matrix" class="Bool (strict)"("Value"=FALSE ("square matrix")) -> ()  [unwired: 2 in, 2 out]
                n3023 = property on="Square pixels" class="Bool (strict)"("Value"=TRUE ("square matrix")) -> ()  [unwired: 2 in, 2 out]
              }
            }
          }
          event "square matrix": Value Change {
            n3024 = event-data() -> ()  [unwired: 1 in, 1 out]
            n3025 = case shown="True" "square matrix" {
              frame False {
              }
              frame True {
                n3026 = property on="square matrix" class="Bool (strict)"("Value"=TRUE ("square matrix")) -> ()  [unwired: 2 in, 2 out]
                n3027 = property on="Square pixels" class="Bool (strict)"("Value"=FALSE ("square matrix")) -> ()  [unwired: 2 in, 2 out]
              }
            }
          }
          event "up", "downright", "down", "downleft", "right", "left", "upright", "upleft": Value Change {
            n3028 = event-data() -> ()  [unwired: 1 in, 6 out]
            n3029 = local read "downright"() -> (w6264:bool)
            n3030 = local read "downleft"() -> (w6266:bool)
            n3031 = local read "upright"() -> (w6262:bool)
            n3032 = local read "upleft"() -> (w6260:bool)
            n3033 = local read "down"() -> (w6265:bool)
            n3034 = local read "right"() -> (w6263:bool)
            n3035 = local read "left"() -> (w6267:bool)
            n3036 = local read "up"() -> (w6261:bool)
            n3037 = Compound Arithmetic op=OR(w6260, w6261, w6262, w6263, w6264, w6265, w6266, w6267) -> (w6259:bool)
            n3038 = case shown="True" w6259 {
              frame False {
              }
              frame True {
                n3039 = stacked-sequence {
                  frame #0 {
                    n3040 = local read "downright"() -> (w6269:bool)
                    n3041 = local read "downleft"() -> (w6271:bool)
                    n3042 = local read "BigSmall"() -> (w6268:bool)
                    n3043 = local read "upright"() -> (w6273:bool)
                    n3044 = local read "upleft"() -> (w6276:bool)
                    n3045 = local read "down"() -> (w6272:bool)
                    n3046 = local read "right"() -> (w6274:bool)
                    n3047 = local read "left"() -> (w6270:bool)
                    n3048 = local read "up"() -> (w6275:bool)
                    n3049 = call "movestageparams.vi"("command"="get") -> ("Params out"=w6279:T20)  [unwired: 1 in]
                    n3050 = Bundle By Name(cluster=w6279, "upleft"=w6276, "up"=w6275, "upright"=w6273, "right"=w6274, "downright"=w6269, "down"=w6272, "downleft"=w6271, "left"=w6270, "Bigsmall"=w6268) -> (w6280:T20)
                    n3051 = call "movestageparams.vi"("Params in"=w6280, "command"="set") -> ()  [unwired: 1 out]
                  }
                  frame #1 {
                    n3052 = disable-structure shown="Disabled" {
                      frame Disabled {
                        n3053 = call "configuration.vi"("command"="get") -> ("config out"=w6283:T11)  [unwired: 2 in, 1 out]
                        n3054 = in-place {
                          n3055 = in-place-cluster #45(w6283) -> ()  [unwired: 2 out]
                          n3056 = in-place-cluster #45("StageL"="StageL", "StageS"="StageS") -> (w6281:T11)
                        }
                        n3057 = call "configuration.vi"("config in"=w6281, "command"="set") -> ()  [unwired: 1 in, 2 out]
                      }
                      frame Enabled {
                      }
                    }
                  }
                  frame #2 {
                    n3058 = call "movestage.vi"() -> ()  [unwired: 12 in]
                  }
                  frame #3 {
                    w6287 = FALSE ("OK Button")
                    w6288 = FALSE ("OK Button")
                    n3059 = property on="down" class="Bool (strict)"("Value"=w6288) -> ()  [unwired: 2 in, 2 out]
                    n3060 = property on="up" class="Bool (strict)"("Value"=w6288) -> ()  [unwired: 2 in, 2 out]
                    n3061 = property on="right" class="Bool (strict)"("Value"=w6288) -> ()  [unwired: 2 in, 2 out]
                    n3062 = property on="left" class="Bool (strict)"("Value"=w6288) -> ()  [unwired: 2 in, 2 out]
                    n3063 = property on="upright" class="Bool (strict)"("Value"=w6287) -> ()  [unwired: 2 in, 2 out]
                    n3064 = property on="downleft" class="Bool (strict)"("Value"=w6287) -> ()  [unwired: 2 in, 2 out]
                    n3065 = property on="downright" class="Bool (strict)"("Value"=w6287) -> ()  [unwired: 2 in, 2 out]
                    n3066 = property on="upleft" class="Bool (strict)"("Value"=w6287) -> ()  [unwired: 2 in, 2 out]
                  }
                }
              }
            }
          }
          event "finite samples": Value Change {
            n3067 = event-data() -> ("NewVal"=w6289:bool)  [unwired: 1 in]
            n3068 = flat-sequence {
              tunnel: w6289 -> [w6290]
              frame #0 {
                n3069 = case shown="True" w6290 {
                  frame False {
                    w6291 = FALSE ("wavdet")
                    n3070 = property on="continuous" class="Bool (strict)"("Value"=TRUE ("continuous for display")) -> ()  [unwired: 2 in, 2 out]
                    n3071 = property on="wavdet" class="Bool (strict)"("Value"=w6291) -> ()  [unwired: 2 in, 2 out]
                    n3072 = property on="save\ndata" class="Bool (strict)"("Value"=w6291) -> ()  [unwired: 2 in, 2 out]
                    n3073 = property on="# of frames" class="DigNum (strict)"("DisabledEnum"=T7."Disabled and Grayed Out" ("Disabled")) -> ()  [unwired: 2 in, 2 out]
                    n3074 = property on="save\ndata" class="Bool (strict)"("DisabledEnum"=T7."Disabled and Grayed Out" ("Disabled")) -> ()  [unwired: 2 in, 2 out]
                    "Save tab" <- enum32{"withsave", "withoutsave"}."withsave" ("Save tab")
                  }
                  frame True {
                    w6298 = FALSE ("continuous for display")
                    n3075 = property on="continuous" class="Bool (strict)"("Value"=w6298) -> ()  [unwired: 2 in, 2 out]
                    n3076 = property on="wavdet" class="Bool (strict)"("Value"=w6298) -> ()  [unwired: 2 in, 2 out]
                    n3077 = local write "Save tab"(enum32{"withsave", "withoutsave"}."withsave" ("Save tab")) -> ()
                    n3078 = property on="save\ndata" class="Bool (strict)"("DisabledEnum"=T7."Enabled" ("Disabled")) -> ()  [unwired: 2 in, 2 out]
